vi "Ambient Sensor Calculations.vi"(9 "PA Voltage":dbl, 10 "RHA Voltage":dbl, 11 "TA Voltage":dbl) -> (1 "PA":dbl, 2 "RHA":dbl, 3 "TA":dbl)   [LabVIEW 2018]
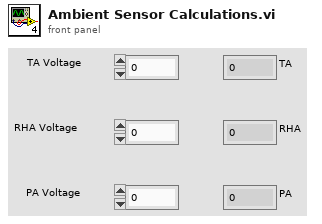
[diagram p1: front panel]
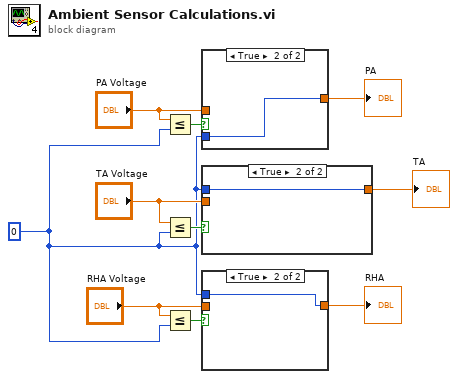
[diagram p0: block diagram]
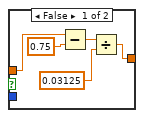
[diagram p2: hidden frame]
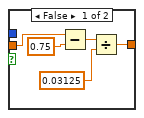
[diagram p3: hidden frame]
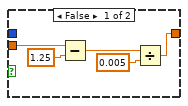
[diagram p4: hidden frame]
diagram:
  w1 = 0
  n1 = Less Or Equal?(x="PA Voltage", y=w1) -> (x <= y?=w7:bool)
  n2 = Less Or Equal?(x="TA Voltage", y=w1) -> (x <= y?=w5:bool)
  n3 = Less Or Equal?(x="RHA Voltage", y=w1) -> (x <= y?=w6:bool)
  n4 = case shown="True" w7 {
    tunnel: "PA Voltage" -> [w15 _]
    tunnel: [w14 w16] -> w10
    tunnel: w1 -> [_ w16]
    frame False {
      n5 = Subtract(x=w15, y=0.75 ("minimum value")) -> (x-y=w12:dbl)
      n6 = Divide(x=w12, y=0.03125 ("minimum value")) -> (x/y=w14:dbl)
    }
    frame True {
    }
  }
  "PA" <- w10
  n7 = case shown="True" w5 {
    tunnel: "TA Voltage" -> [w21 _]
    tunnel: [w20 w22] -> w8
    tunnel: w1 -> [_ w22]
    frame False {
      n8 = Subtract(x=w21, y=1.25 ("minimum value")) -> (x-y=w19:dbl)
      n9 = Divide(x=w19, y=0.005 ("minimum value")) -> (x/y=w20:dbl)
    }
    frame True {
    }
  }
  "TA" <- w8
  n10 = case shown="True" w6 {
    tunnel: "RHA Voltage" -> [w27 _]
    tunnel: [w26 w28] -> w9
    tunnel: w1 -> [_ w28]
    frame False {
      n11 = Subtract(x=w27, y=0.75 ("minimum value")) -> (x-y=w24:dbl)
      n12 = Divide(x=w24, y=0.03125 ("minimum value")) -> (x/y=w26:dbl)
    }
    frame True {
    }
  }
  "RHA" <- w9
